vi "FFT DC抑制(SubVI).vi"(0 "原始訊號":dbl[](array[numeric]), 1 "order":i32, 2 "取樣時間(dt)":dbl, 3 "當下輸入訊號":dbl, 4 "平均參數方式":T1={"averaging mode"=enum."No averaging", "weighting mode"=enum."Exponential", "number of averages"=10} {"number of averages" min=1}) -> (5 "消除DC結果":dbl, 6 "FFT參數":cluster{"f0":dbl, "df":dbl, "magnitude":dbl[]} {"magnitude" format="%.2p"; "f0" format="%0.2p"; "df" format="%0.2p"}, 7 "原始訊號FFT":cluster{"f0":dbl, "df":dbl, "magnitude":dbl[]}(graph))   [LabVIEW 2010]
uses:
  <vilib>/measure/maspectr.llb/FFT Spectrum (Mag-Phase) for 1 Chan.vi
  <vilib>/measure/NI_MAPro.lvlib
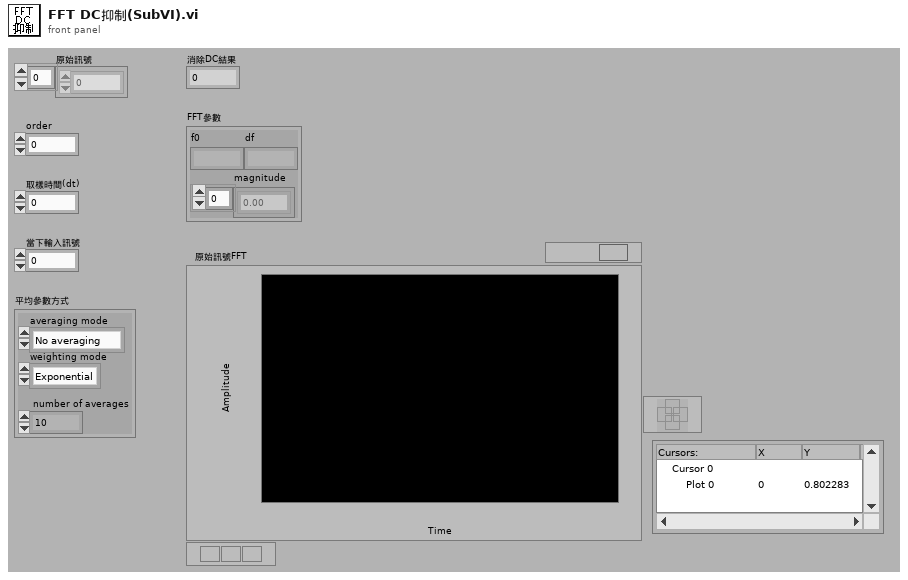
[diagram p1: front panel]
types:
  T1 = cluster{"averaging mode":enum16{"No averaging", "Vector averaging", "RMS averaging", "Peak hold"}, "weighting mode":enum16{"Linear", "Exponential"}, "number of averages":u32}
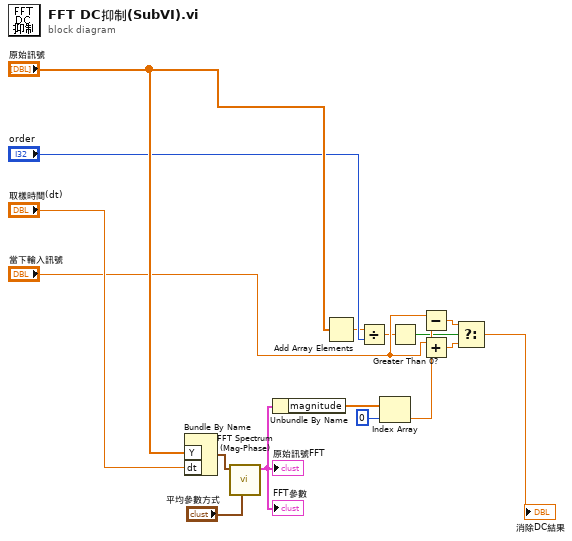
[diagram p0: block diagram]
diagram:
  n1 = Bundle By Name("Y"="原始訊號", "dt"="取樣時間(dt)") -> (w12:waveform(dbl))  [unwired: 1 in]
  n2 = call-poly <vilib>:"FFT Spectrum (Mag-Phase).vi"("averaging parameters"="平均參數方式", "time signal"=w12) -> ("magnitude"=w16:cluster{"f0":dbl, "df":dbl, "magnitude":dbl[]})  [unwired: 5 in, 4 out]
  "原始訊號FFT" <- w16
  "FFT參數" <- w16
  n3 = Unbundle By Name(w16) -> ("magnitude"=w10:dbl[])
  n4 = Add Array Elements(numeric array="原始訊號") -> (sum=w1:dbl)
  n5 = Divide(x=w1, y="order") -> (x/y=w3:dbl)
  n6 = Index Array(array=w10, index=0) -> (element=w15:dbl)
  n7 = Greater Than 0?(x=w3) -> (x > 0?=w4:bool)
  n8 = Subtract(x="當下輸入訊號", y=w15) -> (x-y=w5:dbl)
  n9 = Add(x="當下輸入訊號", y=w15) -> (x+y=w8:dbl)
  n10 = Select(t=w5, s=w4, f=w8) -> (s? t:f=→"消除DC結果":dbl)
